vi "FPGABitfileManager - 9205.vi"(8 "error in (no error)":errorcluster, 10 "Pound in":refnum<class "Pound.lvclass">, 11 "Qbus in":refnum<class "Qbus.lvclass">) -> (0 "error out":errorcluster)   [LabVIEW 2015]
uses:
  <vilib>/addons/Qbus/Qbus.lvclass
  <vilib>/NI/Software Watchdog/Pound/Pound.lvclass
  <vilib>/addons/InsightCM/Devices/Shared/FPGABitfileManager/controls/config.ctl
  <vilib>/FPGAPlugInAG/Dynamic/niLvFpga_Close_Dynamic.vi
  <vilib>/rvi/interface/nirviCloseFPGA/nirviCloseFPGA.xnode
  <vilib>/addons/InsightCM/Devices/Shared/FPGABitfileManager/FPGABitfileManager.lvlib
  <vilib>/addons/InsightCM/Devices/Shared/QbusHelpers/QbusHelper.lvlib
  <vilib>/NI/Software Watchdog/Watchdog/Watchdog.lvclass
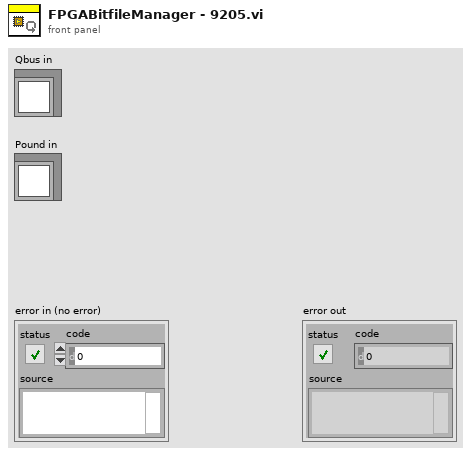
[diagram p1: front panel]
types:
  T1 = typedef "FPGABitfileManager.lvlib/config.ctl" = cluster{"Bitfile reference":refnum<k20>}
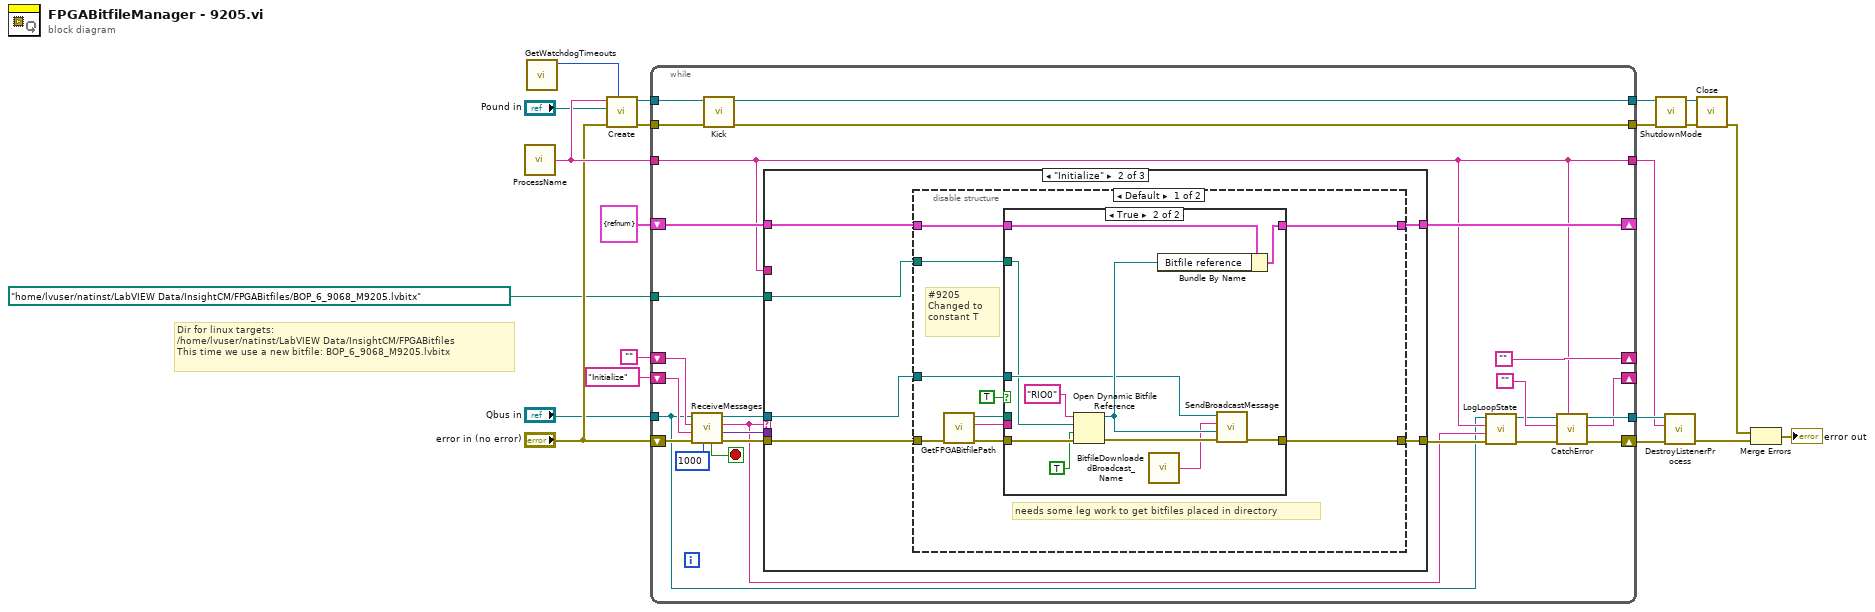
[diagram p0: block diagram]
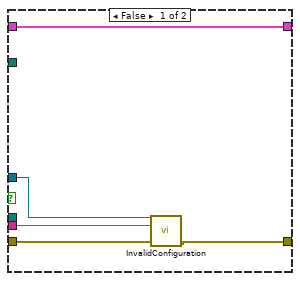
[diagram p3: hidden frame]
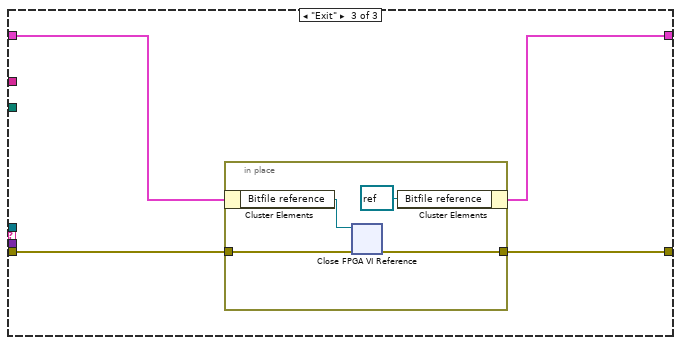
[diagram p5: hidden frame]
diagram:
  # "Dir for linux targets:\n/home/lvuser/natinst/LabVIEW Data/InsightCM/FPGABitfiles\nThis time we use a new bitfile: BOP_6_9068_M9205.lvbitx"
  n1 = call <vilib>:"ProcessName.vi"() -> ("process name"=w15:string)  [unwired: 5 in]
  n2 = call <vilib>:"GetWatchdogTimeouts.vi"() -> ("software timeout"=w2:u32)  [unwired: 10 in, 1 out]
  n3 = call <vilib>:"Create.vi"("Execution Timeout (ms)"=w2, "error in (no error)"="error in (no error)", "Pound"="Pound in", "Name"=w15) -> ("error out"=w9:errorcluster, "Watchdog"=w14:refnum<data-value>)  [unwired: 6 in]
  n4 = while {
    shift-right: [""] -> _
    shift-left: "" -> [w46]
    tunnel: "Qbus in" -> [w26]
    tunnel: w15 -> [w33]
    tunnel: [w37] -> w19
    tunnel: [w33] -> w18
    shift-right: [w35] -> _
    shift-left: "Initialize" -> [w41]
    shift-right: [w39] -> _
    shift-left: T1 {"Bitfile reference"=refnum} ("config") -> [w40]
    tunnel: w14 -> [w32]
    tunnel: [w31] -> w11
    tunnel: w9 -> [w30]
    tunnel: [w28] -> w8
    shift-right: [w38] -> w20
    shift-left: "error in (no error)" -> [w29]
    tunnel: path "/home/lvuser/natinst/LabVIEW Data/InsightCM/FPGABitfiles/BOP_6_9068_M9205.lvbitx" ("Bitfile path") -> [w22]
    stop <- w47 stop-if-true
    n5 = call <vilib>:"ReceiveMessages.vi"("timeout(1000)"=1000 ("Timeout(100)"), "error in (no error)"=w29, "priority action"=w41, "default action"=w46, "Qbus in"=w26) -> ("error out"=w45:errorcluster, "message value"=w42:variant, "action"=w27:string, "Qbus out"=w43:refnum<class "Qbus.lvclass">, "exit"=w47:bool)  [unwired: 2 in]
    n6 = call <vilib>:"Kick.vi"("error in (no error)"=w30, "Watchdog"=w32) -> ("error out"=w28:errorcluster, "Watchdog"=w31:refnum<data-value>)  [unwired: 8 in]
    n7 = case shown="\"Initialize\"" w27 {
      tunnel: w45 -> [w49 w51 w87]
      tunnel: w43 -> [_ w52 _]
      tunnel: [w49 w53 w86] -> w34
      tunnel: w42 -> [_ _ _]
      tunnel: w40 -> [w48 w55 w85]
      tunnel: [w48 w54 w84] -> w39
      tunnel: w33 -> [_ _ _]
      tunnel: w22 -> [_ w50 _]
      frame "", Default {
      }
      frame "Initialize" {
        n8 = disable-structure shown="Default" {
          disable-tunnel: w51 -> [w65 w82]
          disable-tunnel: w55 -> [w64 w83]
          disable-tunnel: [w63 w83] -> w54
          disable-tunnel: [w62 w82] -> w53
          disable-tunnel: w52 -> [w61 _]
          disable-tunnel: w50 -> [w56 _]
          frame condition #0 (active) {
            # "#9205\nChanged to \nconstant T"
            # "needs some leg work to get bitfiles placed in directory"
            n9 = call <vilib>:"GetFPGABitfilePath.vi"("error in (no error)"=w65) -> ("error out"=w59:errorcluster, "description"=w58:string, "fpga bitfile"=w60:path)  [unwired: 7 in, 1 out]
            n10 = case shown="True" TRUE {
              tunnel: w60 -> [_ _]
              tunnel: w59 -> [w69 w80]
              tunnel: [w68 w74] -> w62
              tunnel: w64 -> [w70 w78]
              tunnel: [w70 w77] -> w63
              tunnel: w61 -> [w67 w73]
              tunnel: w58 -> [w66 _]
              tunnel: w56 -> [_ w71]
              frame False {
                n11 = call <vilib>:"InvalidConfiguration.vi"("error in (no error)"=w69, "description"=w66, "Qbus in"=w67) -> ("error out"=w68:errorcluster)  [unwired: 7 in, 1 out]
              }
              frame True {
                n12 = Open Dynamic Bitfile Reference(0:"RIO0" ("Device address"), 1:w71, 2:TRUE ("Run When Loaded"), 3:w80) -> (5:w76:refnum<k20>, 8:w75:errorcluster)  [unwired: 1 in]
                n13 = call <vilib>:"BitfileDownloadedBroadcast_Name.vi"() -> ("message name"=w72:string)  [unwired: 5 in]
                n14 = Bundle By Name(cluster=w78, "Bitfile reference"=w76) -> (w77:T1)
                n15 = call <vilib>:"SendBroadcastMessage.vi"("error in (no error)"=w75, "message value"=w76, "message name"=w72, "Qbus in"=w73) -> ("error in (no error)"=w74:errorcluster)  [unwired: 6 in, 1 out]
              }
            }
          }
          frame condition #1 {
          }
        }
      }
      frame "Exit" {
        n16 = in-place {
          in-place-border: w87 -> [w91]
          in-place-border: [w90] -> w86
          n17 = in-place-cluster #1(w85) -> ("Bitfile reference"=w89:refnum<k20>)
          n18 = xnode "Close FPGA VI Reference"("FPGA VI Reference In"=w89, "error in"=w91) -> ("error out"=w90:errorcluster)
          n19 = in-place-cluster #1("Bitfile reference"=refnum<k20> refnum) -> (w84:T1)
        }
      }
    }
    n20 = call <vilib>:"LogLoopState.vi"("error in (no error)"=w34, "loop action"=w27, "process name"=w33, "Qbus in"=w26) -> ("error out"=w24:errorcluster, "Qbus out"=w23:refnum<class "Qbus.lvclass">)  [unwired: 6 in]
    n21 = call <vilib>:"CatchError.vi"("source"=w33, "error in (no error)"=w24, "next action in"="", "Qbus in"=w23) -> ("error out"=w38:errorcluster, "next action out"=w35:string, "Qbus out"=w37:refnum<class "Qbus.lvclass">)  [unwired: 5 in]
  }
  n22 = call <vilib>:"ShutdownMode.vi"("error in (no error)"=w8, "Watchdog"=w11) -> ("error out"=w10:errorcluster, "Watchdog"=w12:refnum<data-value>)  [unwired: 8 in]
  n23 = call <vilib>:"DestroyListenerProcess.vi"("error in (no error)"=w20, "process name"=w18, "Qbus in"=w19) -> ("error in (no error)"=w7:errorcluster)  [unwired: 7 in, 1 out]
  n24 = call <vilib>:"Close.vi"("error in (no error)"=w10, "Watchdog"=w12) -> ("error out"=w6:errorcluster)  [unwired: 9 in]
  n25 = Merge Errors(w6, w7) -> (→"error out":errorcluster)
